vi "SWERVE DRIVE.vi"(8 "error in (no error)":errorcluster, 11 "controller in":T2) -> (0 "error out":errorcluster, 3 "controller out":T2)   [LabVIEW 2023]
uses:
  ctrl defs/ctrl controllers.ctl
  ctrl defs/ctrl ROTATION SELECT.ctl
  ctrl defs/ctrl DRIVER MODE.ctl
  Global odometry.vi
panel:
  in  "button index\nfor DISABLE\nROTATION":i32=2
  in  "button index\nfor ROTATE":i32=3
  in  "Reset\nFILTER":bool
  in  "apply\nFILTER":bool
  out "Jr":dbl
  in  "button index\nfor TURTLE":i32=1
  in  "button index\nfor TURBO":i32
  in  "button index\nfor STRAFE\nSTEER = OFF":i32=2
  in  "sector width (deg)":dbl(ring)=45.0 format="%#_13g" items=["4-sectors"=90.0, "6-sectors"=60.0, "8-sectors"=45.0, "12-sectors"=30.0, "24-sectors"=15.0, ""=0.0]
  out "Buttons":bool[](array[boolean])
  out "POVs":i16[](array[numeric])
  out "Axes":dbl[](array[numeric])
  in  "select drive controller":T1(ring)=enum."Logitech Extreme 3D Pro"
  in  "notes":string="Joystick 0 - pilot\n\n\"select drive controller\" modifies the X, Y, and twist axis\n\nby default, STRAFE is on and the arc length selected by the control\n\nbutton is momentary STRAFE OFF (usually the driver's thumb)\n\nTURBO and TURTLE added to 0/1  (trigger and thumb)"
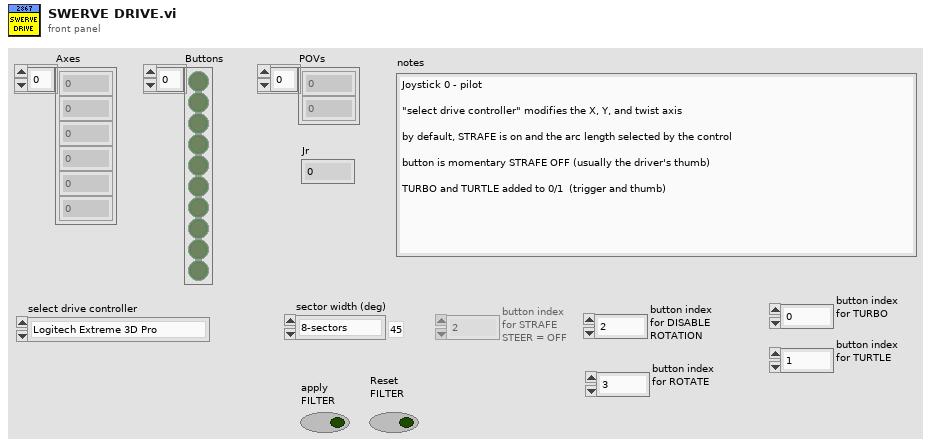
[diagram p1: front panel]
types:
  T1 = enum16{"Logitech Gamepad", "Mad Katz joystick", "Logitech Extreme 3D Pro"}
  T2 = typedef "ctrl controllers.ctl" = cluster{"Axes":dbl[], "Buttons":bool[], "POVs":i16[]}
  T3 = typedef "ctrl ROTATION SELECT.ctl" = enum16{"POV hat ", "TWIST axis"}
  T4 = typedef "ctrl DRIVER MODE.ctl" = enum16{"default", "TURTLE", "TURBO"}
  T5 = enum16{"Left X", "Left Y", "Left trigger", "Right trigger", "Right X", "Right Y"}
  T6 = typedef "ctrl driver input.ctl" = cluster{"Jx":dbl, "Jy":dbl, "Jr ":dbl, "R":dbl, "theta (deg)":dbl, "theta (rad)":dbl, "PARK":bool}
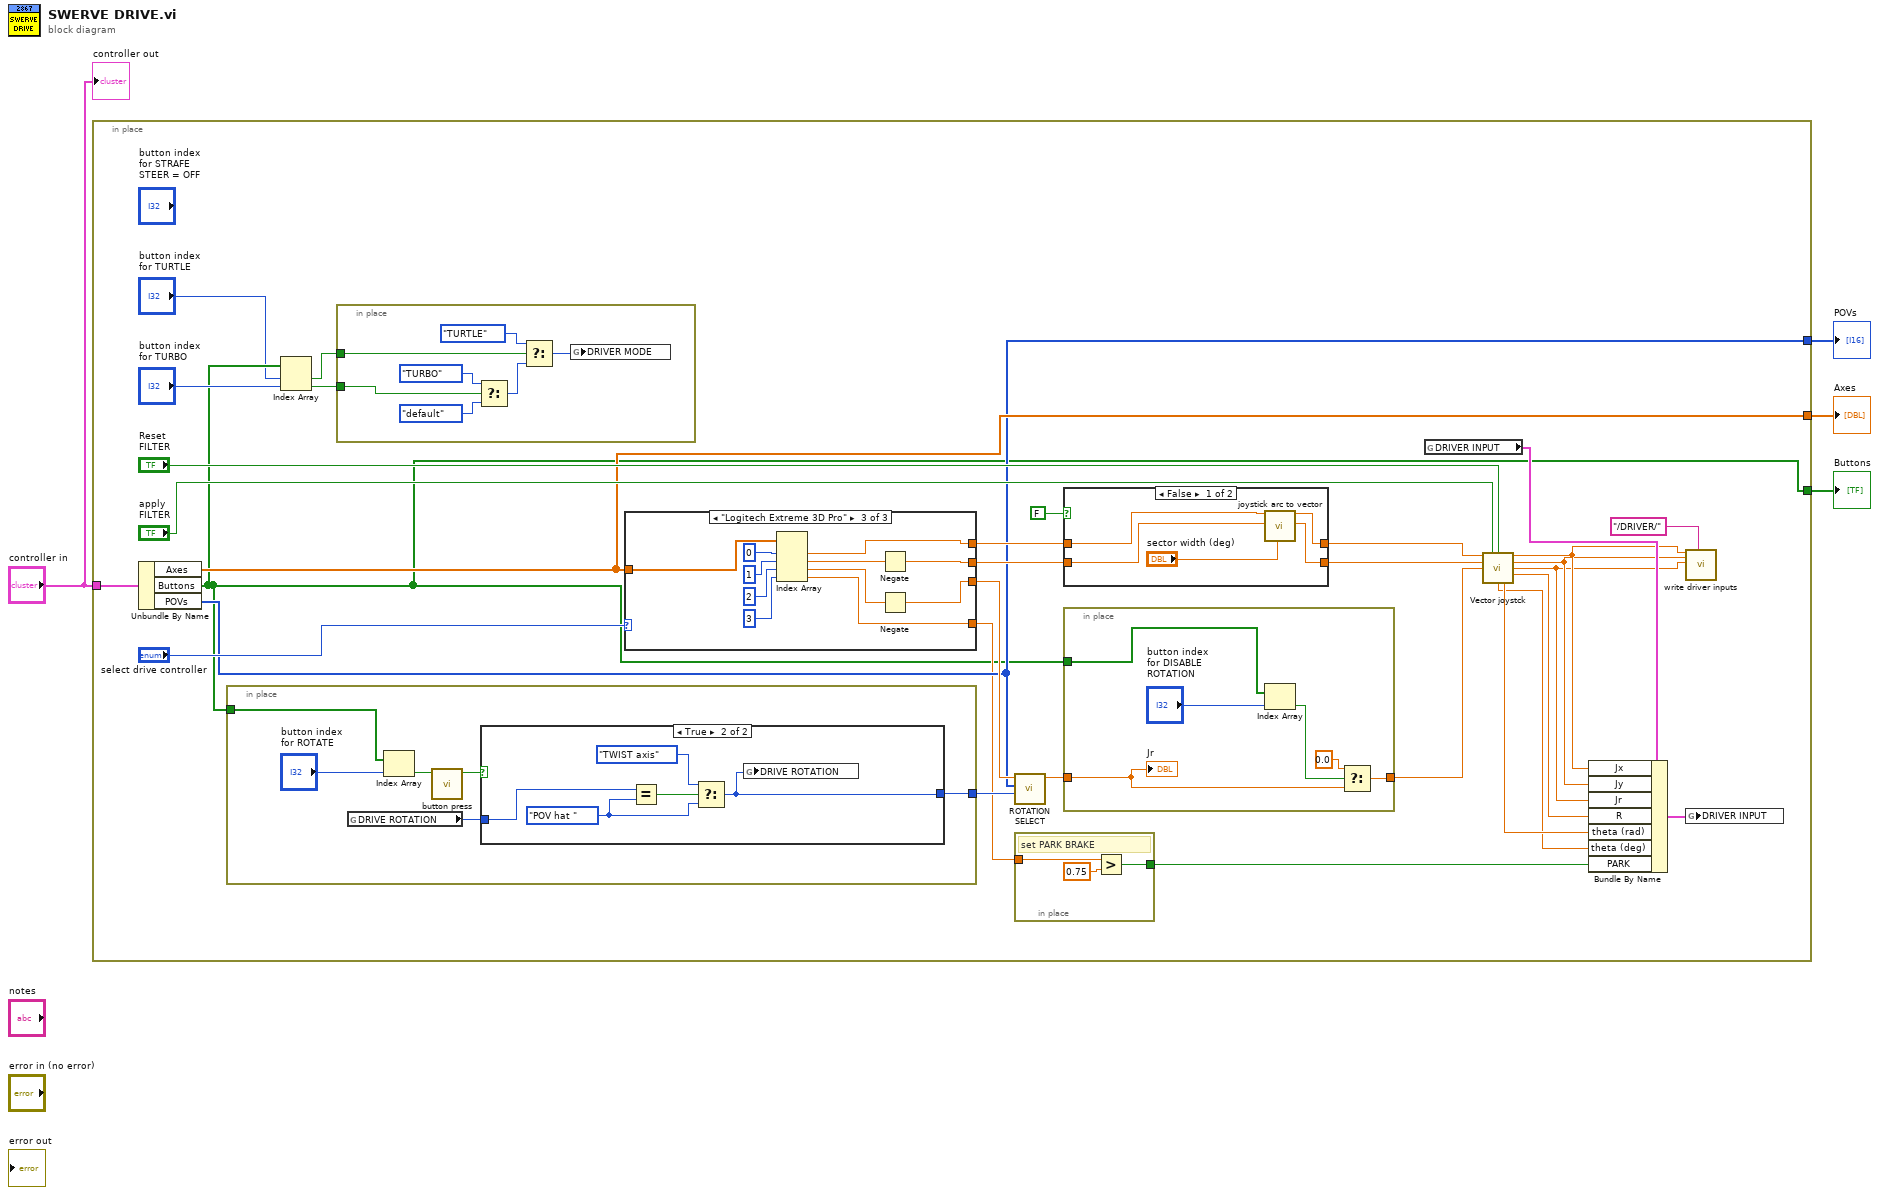
[diagram p0: block diagram]
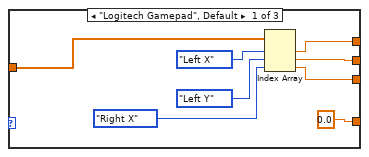
[diagram p4: hidden frame]
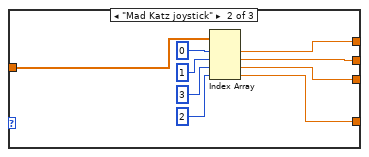
[diagram p5: hidden frame]
diagram:
  n1 = in-place {
    in-place-border: "controller in" -> [w24]
    in-place-border: [w14] -> w3
    in-place-border: [w7] -> w2
    in-place-border: [w13] -> w1
    n2 = Unbundle By Name(w24) -> ("Axes"=w14:dbl[], "Buttons"=w7:bool[], "POVs"=w13:i16[])
    n3 = in-place {
      in-place-border: w7 -> [w50]
      in-place-border: [w46] -> w15
      n4 = global read "Global odometry.vi" "DRIVE ROTATION"() -> (w45:T3)
      n5 = Index Array(array=w50, index="button index\nfor ROTATE") -> (element=w48:bool)
      n6 = call "button press.vi"("button IN"=w48) -> ("Button Pressed?"=w47:bool)  [unwired: 10 in]
      n7 = case shown="True" w47 {
        tunnel: [w51 w55] -> w46
        tunnel: w45 -> [w51 w54]
        frame False {
        }
        frame True {
          w52 = ctrl_ROTATION_SELECT."POV hat " ("ROTATION CONTROL")
          n8 = Equal?(x=w54, y=w52) -> (x = y?=w53:bool)
          n9 = Select(t=ctrl_ROTATION_SELECT."TWIST axis" ("ROTATION CONTROL"), s=w53, f=w52) -> (s? t:f=w55:T3)
          n10 = global write "Global odometry.vi" "DRIVE ROTATION"(w55) -> ()
        }
      }
    }
    n11 = Index Array(array=w7, index #1="button index\nfor TURTLE", index #2="button index\nfor TURBO") -> (element #1=w5:bool, element #2=w18:bool)
    n12 = in-place {
      in-place-border: w5 -> [w63]
      in-place-border: w18 -> [w60]
      n13 = Select(t=ctrl_DRIVER_MODE."TURBO" ("DRIVER MODE"), s=w60, f=ctrl_DRIVER_MODE."default" ("DRIVER MODE")) -> (s? t:f=w61:T4)
      n14 = Select(t=ctrl_DRIVER_MODE."TURTLE" ("DRIVER MODE"), s=w63, f=w61) -> (s? t:f=w57:T4)
      n15 = global write "Global odometry.vi" "DRIVER MODE"(w57) -> ()
    }
    n16 = case shown="\"Logitech Extreme 3D Pro\"" "select drive controller" {
      tunnel: w14 -> [w75 w87 w98]
      tunnel: [w78 w86 w97] -> w21
      tunnel: [w77 w85 w90] -> w20
      tunnel: [w76 w84 w91] -> w31
      tunnel: [0.0 ("upper limit") w79 w88] -> w12
      frame "Logitech Gamepad", Default {
        n17 = Index Array(array=w75, index #1=T5."Left X", index #2=T5."Left Y", index #3=T5."Right X") -> (element #1=w78:dbl, element #2=w77:dbl, element #3=w76:dbl)
      }
      frame "Mad Katz joystick" {
        n18 = Index Array(array=w87, index #1=0 ("index"), index #2=1 ("index"), index #3=3 ("index"), index #4=2 ("index")) -> (element #1=w86:dbl, element #2=w85:dbl, element #3=w84:dbl, element #4=w79:dbl)
      }
      frame "Logitech Extreme 3D Pro" {
        n19 = Index Array(array=w98, index #1=0 ("index"), index #2=1 ("index"), index #3=2 ("index"), index #4=3 ("index")) -> (element #1=w97:dbl, element #2=w96:dbl, element #3=w95:dbl, element #4=w88:dbl)
        n20 = Negate(x=w96) -> (-x=w90:dbl)
        n21 = Negate(x=w95) -> (-x=w91:dbl)
      }
    }
    n22 = call "ROTATION SELECT.vi"("ROTATION CONTROL"=w15, "POVs in"=w13, "TWIST in"=w31) -> ("Jr"=w9:dbl)  [unwired: 8 in]
    n23 = in-place {
      in-place-border: w12 -> [w44]
      in-place-border: [w42] -> w11
      # "set PARK BRAKE"
      n24 = Greater?(x=w44, y=0.75) -> (0:w42:bool)
    }
    n25 = case shown="False" FALSE {
      tunnel: [w68 w70] -> w23
      tunnel: [w67 w69] -> w22
      tunnel: w21 -> [w66 w70]
      tunnel: w20 -> [w65 w69]
      frame False {
        n26 = call "joystick arc to vector.vi"("Jx"=w66, "Jy"=w65, "sector width (deg)"="sector width (deg)") -> ("Jx"=w68:dbl, "Jy"=w67:dbl)  [unwired: 13 in, 2 out]
      }
      frame True {
      }
    }
    n27 = in-place {
      in-place-border: [w41] -> w10
      in-place-border: w9 -> [w40]
      in-place-border: w7 -> [w37]
      n28 = Index Array(array=w37, index="button index\nfor DISABLE\nROTATION") -> (element=w36:bool)
      n29 = Select(t=0.0, s=w36, f=w40) -> (s? t:f=w41:dbl)
      "Jr" <- w40
    }
    n30 = global read "Global odometry.vi" "DRIVER INPUT"() -> (w33:T6)
    n31 = call "Vector joystck.vi"("Jx input"=w23, "apply\nFILTER"="apply\nFILTER", "Reset\nFILTER"="Reset\nFILTER", "Jy input"=w22, "Jr input"=w10) -> ("Jx"=w30:dbl, "Jy"=w29:dbl, "Jr"=w28:dbl, "R"=w27:dbl, "theta (deg)"=w25:dbl, "theta (rad)"=w26:dbl)  [unwired: 5 in]
    n32 = Bundle By Name(cluster=w33, "Jx"=w30, "Jy"=w29, "Jr"=w28, "R"=w27, "theta (rad)"=w26, "theta (deg)"=w25, "PARK"=w11) -> (w32:T6)
    n33 = call "write driver inputs.vi"("Jx"=w30, "Jy"=w29, "Jr"=w28, "stack prefix"="/DRIVER/" ("string")) -> ()  [unwired: 16 in]
    n34 = global write "Global odometry.vi" "DRIVER INPUT"(w32) -> ()
  }
  "Axes" <- w3
  "Buttons" <- w2
  "POVs" <- w1
  "controller out" <- "controller in"
